vi "cRIO-9076_RT.vi"() -> ()   [LabVIEW 2019]
doc: "This VI shows an example of how to implement a closed loop position move using the NI 9505. The position loop is implemented using PID. The output of the loop is used as the command for the current loop, which then sets the PWM duty cycle for the motor. This example assumes that an encoder is connected for position and velocity feedback. This example does not implement advanced motion features such as trajectory generation and splining."
uses:
  <vilib>/LabVIEW Targets/FPGA/cRIO/cRIO-9505/controls.llb/_nicrio_cRIO-9505_DriveStatus.ctl
  <vilib>/Platform/TimedLoop/XDataNode/timing_clust.ctl
  <vilib>/Platform/TimedLoop/XDataNode/nitl_modes.ctl
  <vilib>/Platform/TimedLoop/XDataNode/wakeup.ctl
  <vilib>/FPGAPlugInAG/cRIO-9076/niLvFpga_Open_cRIO-9076.vi
  <vilib>/Utility/error.llb/Error Cluster From Error Code.vi
  <vilib>/rvi/errors/niLvFpgaAdjustHostInterfaceError.vi
  <vilib>/Analysis/3filter.llb/Zero Phase Filter (DBL).vi
  <vilib>/FPGAPlugInAG/cRIO-9076/niLvFpga_Close_cRIO-9076.vi
  <vilib>/rvi/interface/nirviOpenFPGA/nirviOpenFPGA.xnode
  FPGA Bitfiles/gwiz32_FPGATarget2_cRIO-9076FPGA_r3v8jR30hIM.lvbitx
  C:/Program Files (x86)/National Instruments/LabVIEW 2019/Temp/cRIO-9076_FPGA.vi
  <vilib>/rvi/interface/nirviReadWriteControl/nirviReadWriteControl.xnode
  <vilib>/Platform/TimedLoop/XDataNode/XDataNode.xnode
  <vilib>/rvi/interface/nirviCloseFPGA/nirviCloseFPGA.xnode
  <vilib>/Analysis/NI_AALPro.lvlib
  <vilib>/Platform/TimedLoop/XDataNode/XDNodeRunTimeDep.lvlib
  <vilib>/Analysis/NI_AALBase.lvlib
  NiFpgaLv.dll
panel:
  in  "Tab Control":enum32{"Controls", "Plot_data"}(tab)
  out "Saturated?":bool
  in  "samples":i32=10000
  in  "signal type":T1(ring)=enum."square"
  in  "cycles":dbl=1.0 format="%0.2f"
  in  "delay":dbl=180.0 format="%0.2f"
  out "Ball Position (V)":dbl(slide) min=-0.2 max=0.2 step=0.001 scale=0.0..12.0 scale format="%.1f"
  out "Gear Angle Theta (rad)":dbl(knob) scale=-0.8..0.8 scale format="%.2f"
  in  "MANUAL\n/AUTO":bool caption="Auto"
  in  "Motor Voltage 2":dbl(slide) min=-5.0 max=5.0 step=0.01 scale=-6.0..6.0
  out "Motor Voltage":dbl(knob) scale=-6.0..6.0 scale format="%.1f"
  in  "Stiction V \nOffset cw":dbl step=0.01 format="%.4f"
  in  "dc offset":dbl=0.195 format="%.3f"
  in  "amplitude":dbl=0.075 format="%.3f"
  in  "Period(ms)":dbl=50.0 min=0.1 max=1000.0 format="%.2f"
  out "Period OK":bool=TRUE
  in  "STOP":bool
  out "Missed":i16
  in  "Path":path=path "cRIO-9076_RT.vi"
  in  "Stiction V \nOffset ccw":dbl step=0.01 format="%.4f"
  out "RT Plot":cluster{dbl, "ServoAng":dbl, "BallPosn":dbl}(graph)={0.0, "ServoAng"=7.103515625, "BallPosn"=10.50048828125}
  in  "Data plot":bool
  in  "Ball filter":bool=TRUE
  in  "Gear filter":bool=TRUE
  out "Graph":T2(graph)
  out "error out":errorcluster
  # "GWiz v3.2"
  # "Ball & Beam"
  # "Reference\nGenerator"
  # "F2017 2011"
  # "Press Ctrl-H for help"
  # "Export data: right click plot"
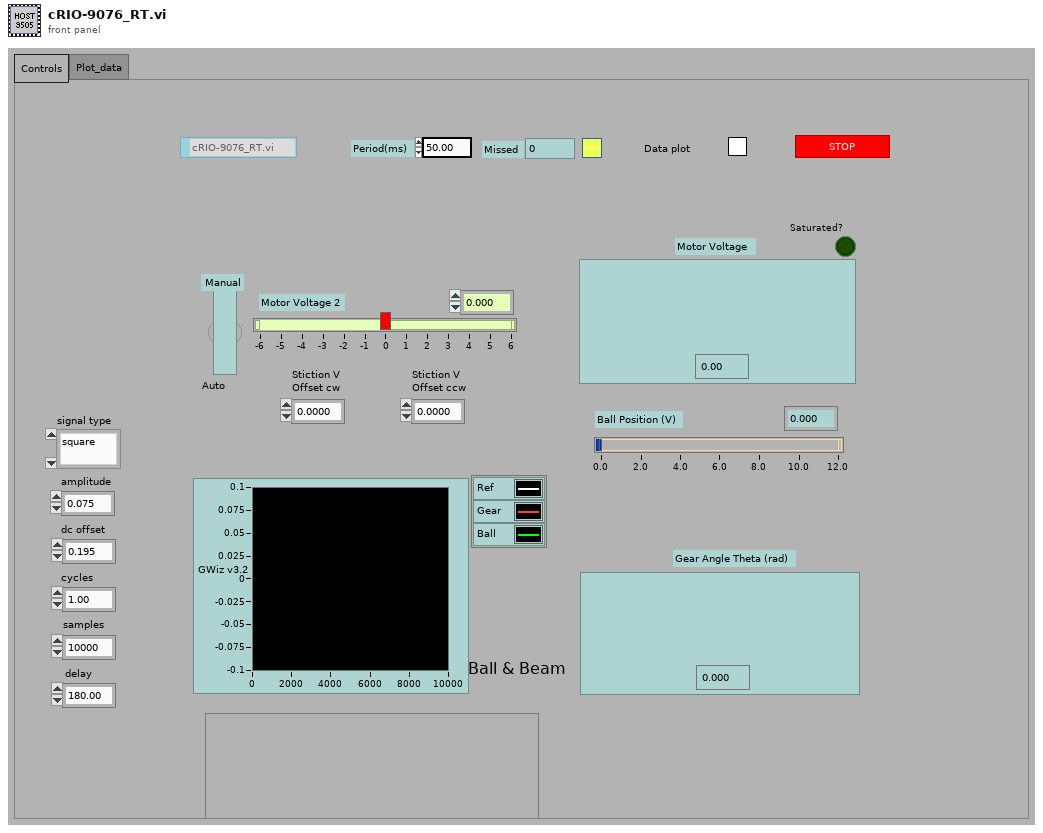
[diagram p1: front panel]
types:
  T1 = enum16{"sine", "cosine", "triangle", "square", "sawtooth", "increasing ramp", "decreasing ramp"}
  T2 = cluster{"Initial time":dbl, dbl, "Data to Plot":dbl[][]}
  T3 = typedef "_nicrio_cRIO-9505_DriveStatus.ctl" = enum8{"Enabled", "Disabled", "Disabled by Drive Fault", "Disabled by Temp. Fault", "Disabled by E-Stop", "Unknown"}
  T4 = typedef "XDNodeRunTimeDep.lvlib/timing_clust.ctl" = cluster{"Expected End [f-1]":u64, "Actual End [f-1]":u64, "Finished Late? [f-1]":bool, "Expected End [i-1]":u64, "Actual End [i-1]":u64, "Finished Late? [i-1]":bool, "Expected Start [i]":u64, "Actual Start [i]":u64, "Expected Start [f]":u64, "Actual Start [f]":u64, "Source Name":string, "Structure Name":string, "Period":i64, "Deadline":i64, "Offset":i64, "Start":i64, "Priority":i32, "Timeout":i32, "Mode":T5, "Wakeup Reason":T6, "Error":errorcluster, "Source Type":string, "Secondary Source Type":string, "Global End Time":u64, "Global Start Time":u64, "Frame Duration":u64, "Iteration Duration":u64, "Assigned CPU":i32, "I/O Scan Engine Mode":u32}
  T5 = typedef "XDNodeRunTimeDep.lvlib/nitl_modes.ctl" = enum32{"No Change", "Process missed periods, maintain original phase", "Discard missed periods, maintain original phase", "Process missed periods, ignore original phase", "Discard missed periods, ignore original phase"}
  T6 = typedef "XDNodeRunTimeDep.lvlib/wakeup.ctl" = enum32{"Normal", "Aborted", "Asynchronous wakeup", "Timing source error", "Timed loop error", "Timeout"}
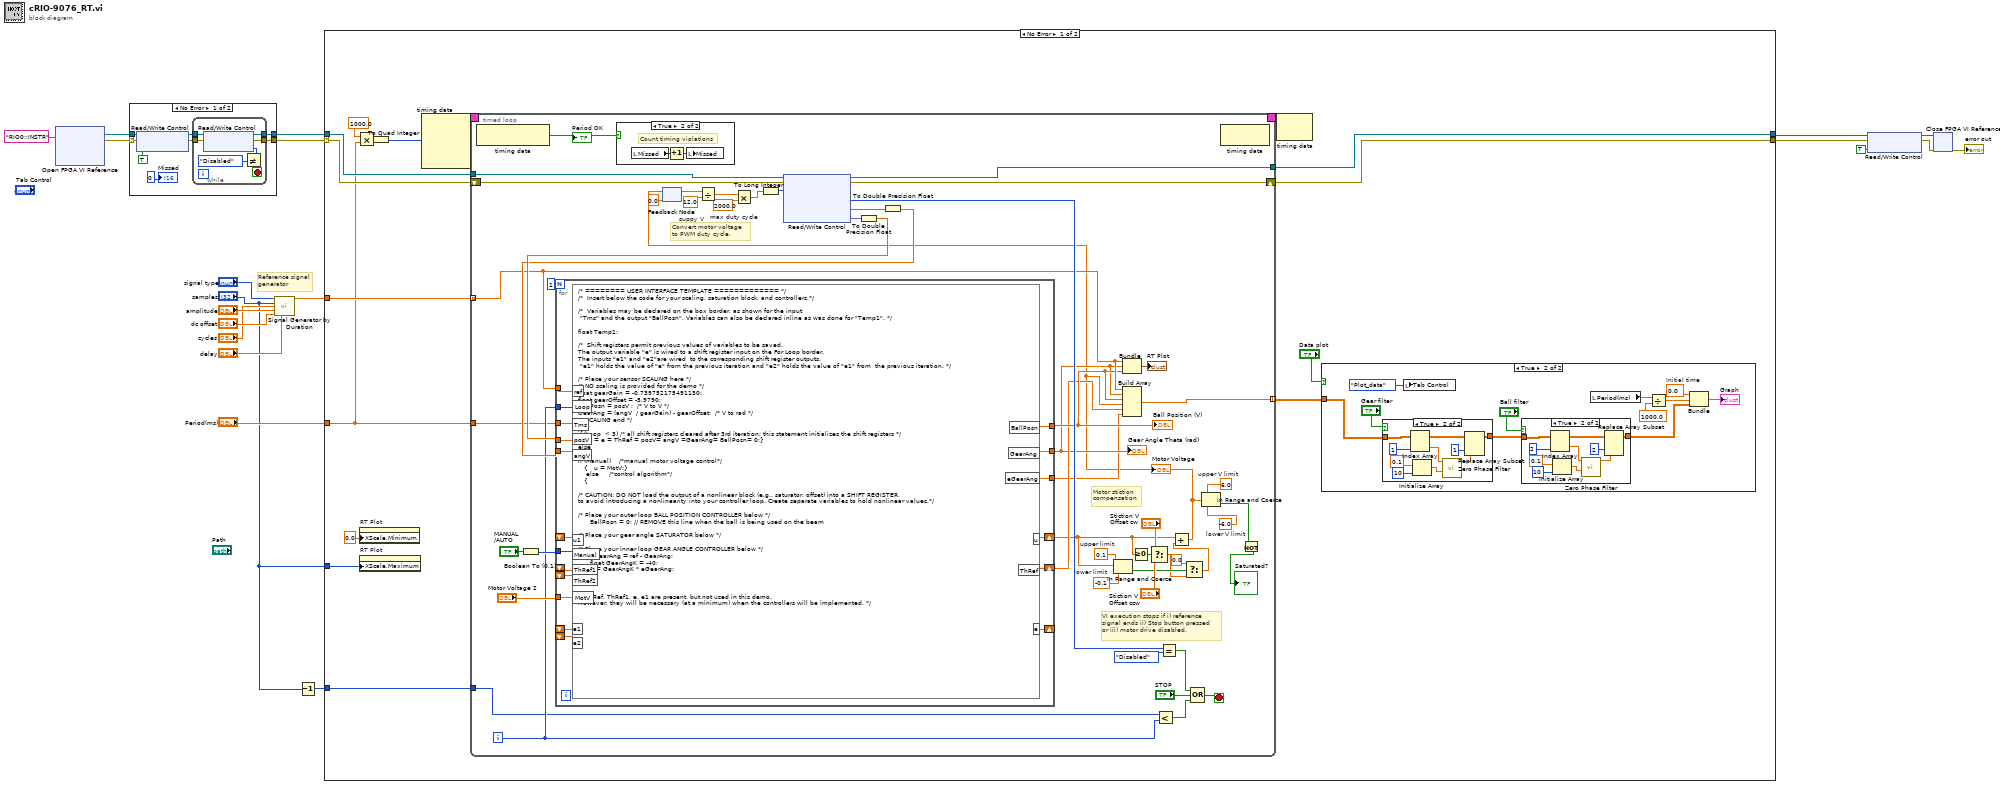
[diagram p0: block diagram]
diagram:
  # "Reference signal\ngenerator"
  n1 = xnode "Open FPGA VI Reference"("resource name"="RIO0::INSTR") -> ("FPGA VI Reference Out"=w7:refnum<k20>, "error out"=w14:errorcluster)  [unwired: 1 in]
  n2 = case shown="No Error" w14 {
    selector: w14 -> [w23 w36]
    tunnel: w7 -> [w26 w37]
    tunnel: [w28 w37] -> w15
    tunnel: [w22 w36] -> w13
    frame No Error {
      n3 = xnode "Read/Write Control"("FPGA VI Reference In"=w26, "error in"=w23, "Enable Drive"=TRUE) -> ("FPGA VI Reference Out"=w25:refnum<k20>, "error out"=w24:errorcluster)
      n4 = while {
        tunnel: [w35] -> w28
        tunnel: w25 -> [w31]
        tunnel: w24 -> [w32]
        tunnel: [w29] -> w22
        stop <- w30 stop-if-true
        n5 = xnode "Read/Write Control"("FPGA VI Reference In"=w31, "error in"=w32) -> ("FPGA VI Reference Out"=w35:refnum<k20>, "error out"=w29:errorcluster, "Drive Status"=w34:T3)
        n6 = Not Equal?(x=w34, y=_nicrio_cRIO-9505_DriveStatus."Disabled") -> (x != y?=w30:bool)
      }
      "Missed" <- i16 0 ("Missed")
    }
    frame Error {
      # "Error occurred. Do not run."
    }
  }
  n7 = call <vilib>:"Signal Generator by Duration.vi"("signal type"="signal type", "# of samples"="samples", "frequency"="cycles", "amplitude"="amplitude", "dc offset"="dc offset", "phase in"="delay") -> ("signal"=w9:dbl[])  [unwired: 6 in, 3 out]
  n8 = Decrement(x="samples") -> (x-1=w2:i32)
  n9 = case shown="No Error" w13 {
    selector: w13 -> [w51 w163]
    tunnel: w15 -> [w53 w164]
    tunnel: [w42 w164] -> w20
    tunnel: [w52 w163] -> w19
    tunnel: w9 -> [w50 _]
    tunnel: w2 -> [w49 _]
    tunnel: "Period(ms)" -> [w46 _]
    tunnel: "samples" -> [w38 _]
    frame No Error {
      n10 = Multiply(x=1000.0, y=w46) -> (x*y=w44:dbl)
      n11 = property on="RT Plot" class="WFChart (strict)"("XScale.Minimum"=0.0 ("X Scale.Range:Minimum")) -> ()  [unwired: 2 in, 2 out]
      n12 = property on="RT Plot" class="WFChart (strict)"("XScale.Maximum"=w38) -> ()  [unwired: 2 in, 2 out]
      n13 = To Quad Integer(1:w44) -> (0:w43:i64)
      n14 = node-c288(w43) -> (w48:T4)  [unwired: 3 in]
      n15 = timed-loop {
        tunnel: w53 -> [w135]
        tunnel: [w133] -> w42
        shift-right: [w132] -> w52
        shift-left: w51 -> [w134]
        tunnel: w50 -> [w106] mode=indexing
        tunnel: w49 -> [w108]
        tunnel: w46 -> [w102]
        timing: w48 -> [_]
        timing-out: [_] -> w47
        tunnel: [w103] -> w41 mode=indexing
        i -> [w109]
        stop <- w129 stop-if-true
        w88 = -6.0  # lower V limit
        w89 = 6.0  # upper V limit
        w95 = -0.1  # lower limit
        w96 = 0.1  # upper limit
        w114 = 2000.0  # max duty cycle
        w113 = 12.0  # suppy V
        # "Convert motor voltage\nto PWM duty cycle."
        # "VI execution stops if i) reference\nsignal ends ii) Stop button pressed\nor iii) motor drive disabled."
        # "Motor stiction\ncompensation"
        n16 = node-c288() -> (w116:bool)  [unwired: 1 in]
        "Period OK" <- w116
        n17 = Boolean To (0,1)(Boolean="MANUAL\n/AUTO") -> (0, 1=w121:i16)
        n18 = case shown="True" w116 {
          frame False {
          }
          frame True {
            # "Count timing violations"
            n19 = local read "Missed"() -> (w137:i16)
            n20 = Increment(x=w137) -> (x+1=w136:i16)
            n21 = local write "Missed"(w136) -> ()
          }
        }
        n22 = feedback #1(0.0) -> (w111:dbl)
        n23 = Divide(x=w111, y=w113) -> (x/y=w112:dbl)
        n24 = Multiply(x=w112, y=w114) -> (x*y=w110:dbl)
        n25 = To Long Integer(number=w110) -> (32bit integer=w107:i32)
        n26 = xnode "Read/Write Control"("FPGA VI Reference In"=w135, "error in"=w134, "Position Setpoint"=w107) -> ("FPGA VI Reference Out"=w133:refnum<k20>, "error out"=w132:errorcluster, "Drive Status"=w131:T3, "Gear Pot"=w127:fxp<+/-,16,5>, "Ball Pot"=w126:fxp<+/-,16,5>)
        n27 = To Double Precision Float(number=w126) -> (double precision float=w124:dbl)
        n28 = To Double Precision Float(number=w127) -> (double precision float=w119:dbl)
        n29 = for {
          N: 1 -> [_]
          tunnel: w106 -> [w158]
          tunnel: w124 -> [w157]
          shift-right: [w143] -> w94
          shift-left: _ -> [w156]
          shift-right: [w155] -> _
          shift-left: _ -> [w154]
          tunnel: [w153] -> w105
          tunnel: w102 -> [w152]
          tunnel: w119 -> [w151]
          tunnel: [w150] -> w101
          tunnel: w121 -> [w149]
          tunnel: "Motor Voltage 2" -> [w148]
          shift-right: [w147] -> w104
          shift-left: _ -> [w146]
          shift-left: _ -> [w145]
          tunnel: w109 -> [w144]
          shift-left: _ -> [w142]
          tunnel: [w141] -> w90
          n30 = formula code="/* ======== USER INTERFACE TEMPLATE ============= */\n/*  Insert below the code for your scaling, saturation block, and controllers.*/\n\n/*  Variables may be declared on the box border, as shown for the input \n \"Tms\" and the output \"BallPosn\". Variables can also be declared inline as was done for \"Temp1\". */\n\nfloat Temp1; \n\n/*  Shift registers permit previous values of variables to be saved. \nThe output variable \"e\" is wired to a shift register input on the For Loop border.  \nThe inputs \"e1\" and \"e2\"are wired  to the corresponding shift register outputs.\n \"e1\" holds the value of \"e\" from the previous iteration and \"e2\" holds the value of \"e1\" from  the previous iteration. */\n\n/* Place your sensor SCALING here */\n/* NO scaling is provided for the demo */\nfloat gearGain = -0.739752175491130;\nfloat gearOffset = -5.9790;\nBallPosn = posV ;  /* V to V */\nGearAng = (angV  / gearGain) - gearOffset;  /* V to rad */\n/* SCALING end */\n\nif (Loop  < 3) /* all shift registers cleared after 3rd iteration; this statement initializes the shift registers */\n   {u = e = ThRef = posV= angV =GearAng= BallPosn= 0;}\nelse\n{\nif (Manual)    /*manual motor voltage control*/\n   {   u = MotV;}\n    else     /*control algorithm*/\n   { \n\n/* CAUTION: DO NOT load the output of a nonlinear block (e.g., saturator, offset) into a SHIFT REGISTER, \nto avoid introducing a nonlinearity into your controller loop. Create separate variables to hold nonlinear values.*/\n\n/* Place your outer loop BALL POSITION CONTROLLER below */\n      BallPosn = 0; // REMOVE this line when the ball is being used on the beam\n\n/* Place your gear angle SATURATOR below */\n\n/* Place your inner loop GEAR ANGLE CONTROLLER below */\n      eGearAng = ref - GearAng;\n      float GearAngK = -40;\n      u = GearAngK * eGearAng;\n   }\n} \n    \n/* ThRef, ThRef1, e, e1 are present, but not used in this demo.  \nHowever, they will be necessary (at a minimum) when the controllers will be implemented. */"("Tms"=w152, "Loop"=w144, "u1"=w156, "e1"=w154, "ref"=w158, "posV"=w157, "angV"=w151, "Manual"=w149, "MotV"=w148, "ThRef1"=w146, "e2"=w145, "ThRef2"=w142) -> ("u"=w143:dbl, "e"=w155:dbl, "BallPosn"=w153:dbl, "GearAng"=w150:dbl, "ThRef"=w147:dbl, "eGearAng"=w141:dbl)
        }
        "Ball Position (V)" <- w105
        "Gear Angle Theta (rad)" <- w101
        n31 = In Range and Coerce(upper limit=w96, x=w94, lower limit=w95) -> (In Range?=w93:bool)  [unwired: 1 out]
        n32 = Bundle(w106, "GearAng"=w101, "BallPosn"=w105) -> (→"RT Plot":cluster{dbl, "GearAng":dbl, "BallPosn":dbl})  [unwired: 1 in]
        n33 = Greater Or Equal To 0?(x=w94) -> (x >= 0?=w118:bool)
        n34 = Select(t="Stiction V \nOffset cw", s=w118, f="Stiction V \nOffset ccw") -> (s? t:f=w92:dbl)
        n35 = Less?(x=w108, y=w109) -> (x < y?=w120:bool)
        n36 = Equal?(x=w131, y=_nicrio_cRIO-9505_DriveStatus."Disabled") -> (x = y?=w128:bool)
        n37 = Select(t=0.0, s=w93, f=w92) -> (s? t:f=w99:dbl)
        n38 = Add(x=w94, y=w99) -> (x+y=w87:dbl)
        "Motor Voltage" <- w87
        n39 = feedback-in #1(w87) -> ()
        n40 = Build Array(w106, w101, w105, w87, w104, w90) -> (w103:dbl[])
        n41 = Compound Arithmetic op=OR(w128, "STOP", w120) -> (w129:bool)
        n42 = In Range and Coerce(upper limit=w89, x=w87, lower limit=w88) -> (In Range?=w86:bool)  [unwired: 1 out]
        n43 = node-c288() -> ()  [unwired: 1 in, 1 out]
        n44 = Not(x=w86) -> (.not. x?=→"Saturated?":bool)
      }
      n45 = node-c288(w47) -> ()  [unwired: 1 out]
      n46 = case shown="True" "Data plot" {
        tunnel: w41 -> [_ w59]
        frame False {
        }
        frame True {
          w64 = 0.0  # Initial time
          n47 = case shown="True" "Gear filter" {
            tunnel: w59 -> [w75 w77]
            tunnel: [w75 w76] -> w61
            frame False {
            }
            frame True {
              n48 = Index Array(array=w77, index (col)=1 ("index (row)")) -> (element=w79:dbl[])  [unwired: 1 in]
              n49 = Initialize Array(0.1 ("element"), 10 ("dimension size")) -> (w82:dbl[])
              n50 = call-poly <vilib>:"Zero Phase Filter.vi"("Forward Coefficients"=w82, "X"=w79) -> ("Filtered X"=w78:dbl[])  [unwired: 8 in, 1 out]
              n51 = Replace Array Subset(array=w77, new element=w78, index (col)=1 ("disabled index (col)")) -> (w76:dbl[][])  [unwired: 1 in]
            }
          }
          n52 = local write "Tab Control"(enum32{"Controls", "Plot_data"}."Plot_data" ("Tab Control")) -> ()
          n53 = case shown="True" "Ball filter" {
            tunnel: w61 -> [w65 w67]
            tunnel: [w65 w66] -> w60
            frame False {
            }
            frame True {
              n54 = Index Array(array=w67, index (col)=2 ("index (row)")) -> (element=w69:dbl[])  [unwired: 1 in]
              n55 = Initialize Array(0.1 ("element"), 10 ("dimension size")) -> (w72:dbl[])
              n56 = call-poly <vilib>:"Zero Phase Filter.vi"("Forward Coefficients"=w72, "X"=w69) -> ("Filtered X"=w68:dbl[])  [unwired: 8 in, 1 out]
              n57 = Replace Array Subset(array=w67, new element=w68, index (col)=2 ("disabled index (col)")) -> (w66:dbl[][])  [unwired: 1 in]
            }
          }
          n58 = local read "Period(ms)"() -> (w58:dbl)
          n59 = Divide(x=w58, y=1000.0) -> (x/y=w62:dbl)
          n60 = Bundle("Initial time"=w64, w62, w60) -> (→"Graph":cluster{"Initial time":dbl, dbl, dbl[][]})  [unwired: 1 in]
        }
      }
    }
    frame Error {
      # "Error occurred. Do not run."
    }
  }
  n61 = xnode "Read/Write Control"("FPGA VI Reference In"=w20, "error in"=w19, "Disable Drive"=TRUE) -> ("FPGA VI Reference Out"=w18:refnum<k20>, "error out"=w17:errorcluster)
  n62 = xnode "Close FPGA VI Reference"("FPGA VI Reference In"=w18, "error in"=w17) -> ("error out"=→"error out":errorcluster)
